vi "referfencesize.vi"(2 "Digital waveforms in":digitalwaveform[](array[waveform]), 3 "Analog waveforms in":waveform(dbl)[](array[waveform]), 4 "reference waveforms to":string) -> (1 "number of samples":i32)   [LabVIEW 2015]
uses:
  <vilib>/Waveform/DWDTOps.llb/DWDT Digital Size.vi
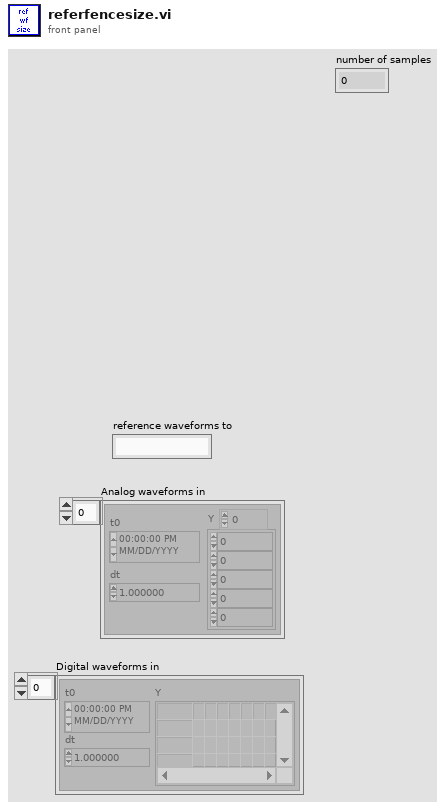
[diagram p1: front panel]
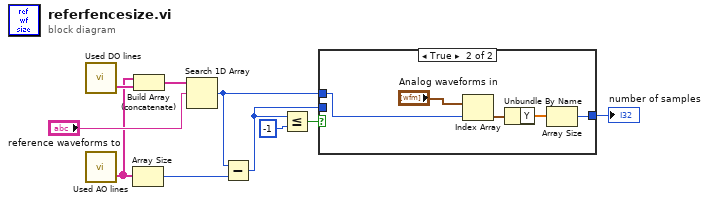
[diagram p0: block diagram]
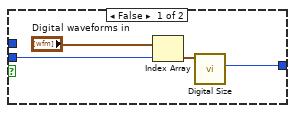
[diagram p2: hidden frame]
diagram:
  n1 = call "Used DO lines.vi"() -> ("used DO names"=w9:string[])  [unwired: 2 in, 1 out]
  n2 = call "Used AO lines.vi"() -> ("used AO names"=w7:string[])  [unwired: 2 in, 1 out]
  n3 = Array Size(array=w7) -> (size(s)=w5:i32)
  n4 = Build Array (concatenate)(w7, w9) -> (w8:string[])
  n5 = Search 1D Array(1D array=w8, element="reference waveforms to") -> (index of element=w2:i32)  [unwired: 1 in]
  n6 = Subtract(x=w2, y=w5) -> (x-y=w3:i32)
  n7 = Less Or Equal?(x=w3, y=-1) -> (x <= y?=w4:bool)
  n8 = case shown="True" w4 {
    tunnel: w3 -> [w14 _]
    tunnel: [w12 w16] -> w1
    tunnel: w2 -> [_ w17]
    frame False {
      n9 = Index Array(array="Digital waveforms in", index=w14) -> (element=w13:digitalwaveform)
      n10 = call-poly <vilib>:"Digital Size.vi"("digital waveform in"=w13) -> ("number of samples"=w12:i32)  [unwired: 7 in, 3 out]
    }
    frame True {
      n11 = Index Array(array="Analog waveforms in", index=w17) -> (element=w19:waveform(dbl))
      n12 = Unbundle By Name(w19) -> ("Y"=w18:dbl[])
      n13 = Array Size(array=w18) -> (size(s)=w16:i32)
    }
  }
  "number of samples" <- w1
